vi "PNA_display_mag_phase.vi"(0 "VISA resource name":refnum<visa-resource-name>, 1 "Channel (1)":i32=1, 2 "Measurement Name (CH1_S11)":string="CH1_S11_1", 3 "error in (no error)":errorcluster, 4 "Display format 1-2":T1 {"Display Format 1" items=["Magnitude Linear", "Magnitude Logarithmic", "Phase", "Unwrapped phase", "Imaginary", "Real", "Polar", "Smith Chart", "Smith Admittance", "SWR", "Group Delay", "Kelvin", "Fahrenheit", "Celsius"]; "Display Format 2" items=["Magnitude Linear", "Magnitude Logarithmic", "Phase", "Unwrapped phase", "Imaginary", "Real", "Polar", "Smith Chart", "Smith Admittance", "SWR", "Group Delay", "Kelvin", "Fahrenheit", "Celsius"]}) -> (5 "VISA resource name out":refnum<visa-resource-name>, 6 "Cluster":cluster{"Magnitude":dbl[], "Phase":dbl[]}, 7 "error out":errorcluster)   [LabVIEW 2020]
uses:
  <instrlib>/Keysight PNA Series/Keysight PNA Series.lvlib
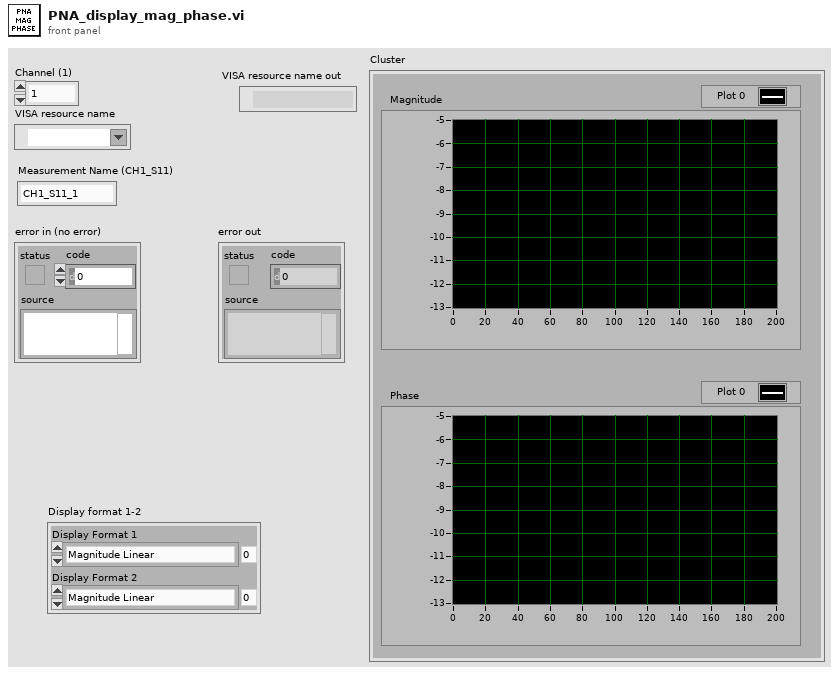
[diagram p1: front panel]
types:
  T1 = cluster{"Display Format 2":i32, "Display Format 1":i32}
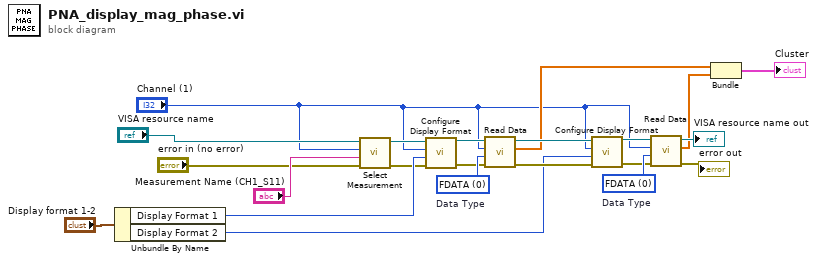
[diagram p0: block diagram]
diagram:
  w19 = 0 items=["FDATA", "RDATA", "SDATA", "FMEM", "SMEM", "SDIV"]  # Data Type
  w22 = 0 items=["FDATA", "RDATA", "SDATA", "FMEM", "SMEM", "SDIV"]  # Data Type
  n1 = Unbundle By Name("Display format 1-2") -> ("Display Format 1"=w8:i32, "Display Format 2"=w7:i32)
  n2 = call <instrlib>:"Select Measurement.vi"("error in (no error)"="error in (no error)", "Measurement Name (CH1_S11_1)"="Measurement Name (CH1_S11)", "Channel (1)"="Channel (1)", "VISA resource name"="VISA resource name") -> ("error out"=w6:errorcluster, "VISA resource name out"=w5:refnum<visa-resource-name>)  [unwired: 6 in]
  n3 = call <instrlib>:"Configure Display Format.vi"("error in (no error)"=w6, "Display Format (0: Magnitude Linear)"=w8, "Channel (1)"="Channel (1)", "VISA resource name"=w5) -> ("error out"=w21:errorcluster, "VISA resource name out"=w20:refnum<visa-resource-name>)  [unwired: 6 in]
  n4 = call <instrlib>:"Read Data.vi"("error in (no error)"=w21, "Data Type (0: FDATA)"=w22, "Channel (1)"="Channel (1)", "VISA resource name"=w20) -> ("error out"=w15:errorcluster, "Data"=w12:dbl[], "VISA resource name out"=w16:refnum<visa-resource-name>)  [unwired: 5 in]
  n5 = call <instrlib>:"Configure Display Format.vi"("error in (no error)"=w15, "Display Format (0: Magnitude Linear)"=w7, "Channel (1)"="Channel (1)", "VISA resource name"=w16) -> ("error out"=w18:errorcluster, "VISA resource name out"=w17:refnum<visa-resource-name>)  [unwired: 6 in]
  n6 = call <instrlib>:"Read Data.vi"("error in (no error)"=w18, "Data Type (0: FDATA)"=w19, "Channel (1)"="Channel (1)", "VISA resource name"=w17) -> ("error out"=→"error out":errorcluster, "Data"=w11:dbl[], "VISA resource name out"=→"VISA resource name out":refnum<visa-resource-name>)  [unwired: 5 in]
  n7 = Bundle("Data"=w12, "Data"=w11) -> (→"Cluster":cluster{"Data":dbl[], "Data":dbl[]})  [unwired: 1 in]
